vi "Stop.vi"(0 "SystemEvents in":refnum<class "SystemEvents.lvclass">, 1 "event data":variant, 5 "error in (no error)":errorcluster) -> (14 "SystemEvents out":refnum<class "SystemEvents.lvclass">, 19 "error out":errorcluster)   [LabVIEW 2017, in "SystemEvents.lvclass"]
doc: "Fires the Stop event."
uses:
  SystemEvents.lvclass
  SystemEvents.lvclass/SystemEvents.ctl
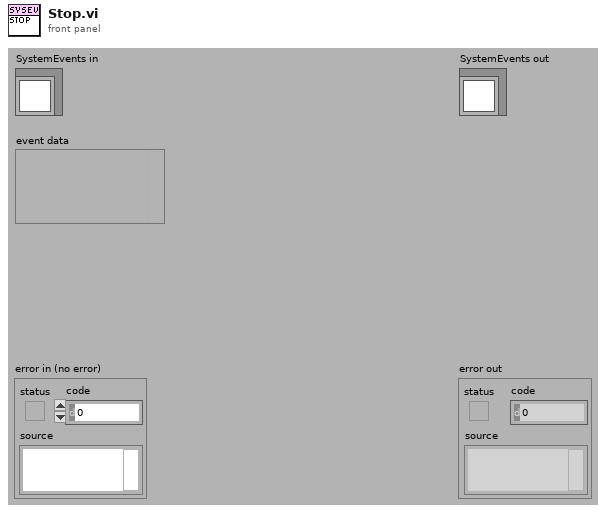
[diagram p1: front panel]
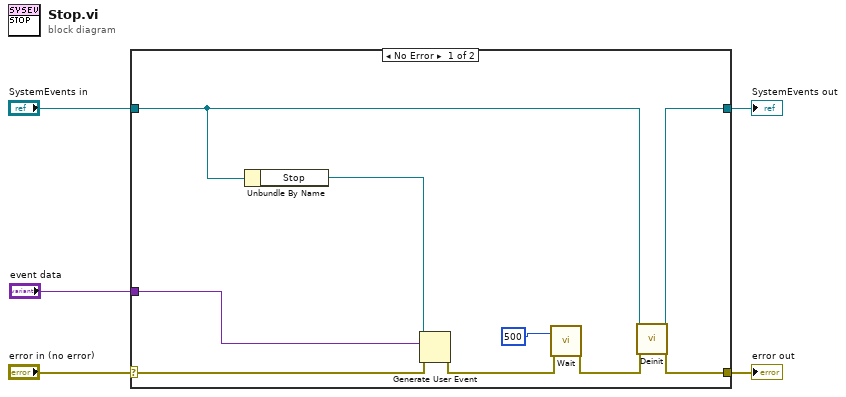
[diagram p0: block diagram]
diagram:
  n1 = case shown="No Error" "error in (no error)" {
    selector: "error in (no error)" -> [w14 w16]
    tunnel: [w8 w16] -> w4
    tunnel: [w7 w15] -> w2
    tunnel: "SystemEvents in" -> [w6 w15]
    tunnel: "event data" -> [w12 _]
    frame No Error {
      n2 = Unbundle By Name(w6) -> ("Stop"=w13:refnum<user-event>)
      n3 = Generate User Event(user event=w13, event data cluster=w12, error in=w14) -> (error out=w10:errorcluster)  [unwired: 1 in, 1 out]
      n4 = call "Wait.vi"("milliseconds to wait"=u32 500, "error in (no error)"=w10) -> ("error out"=w9:errorcluster)  [unwired: 17 out]
      n5 = call-dynamic "Deinit.vi"("SystemEvents in"=w6, "error in (no error)"=w9) -> ("SystemEvents out"=w7:refnum<class "SystemEvents.lvclass">, "error out"=w8:errorcluster)  [unwired: 16 out]
    }
    frame Error {
    }
  }
  "error out" <- w4
  "SystemEvents out" <- w2
